vi "Pose_Create.vi"(9 "Heading":dbl, 10 "Y":dbl, 11 "X":dbl) -> (3 "out POSe":T1)   [LabVIEW 2019, in "PathExecution_Library.lvlib"]
uses:
  PathExecution_Library.lvlib
  POSE.ctl
  TRANSLATION.ctl
  ROTATION.ctl
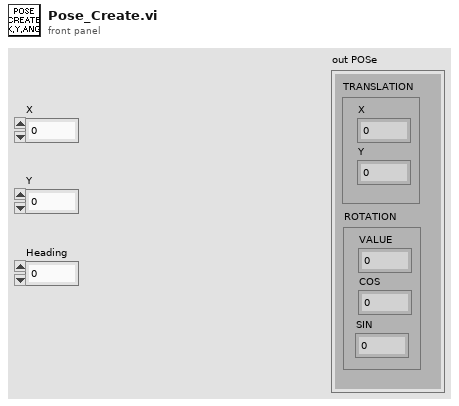
[diagram p1: front panel]
types:
  T1 = typedef "PathExecution_Library.lvlib/POSE.ctl" = cluster{"TRANSLATION":T2, "ROTATION":T3}
  T2 = typedef "PathExecution_Library.lvlib/TRANSLATION.ctl" = cluster{"X":dbl, "Y":dbl}
  T3 = typedef "PathExecution_Library.lvlib/ROTATION.ctl" = cluster{"VALUE":dbl, "COS":dbl, "SIN":dbl}
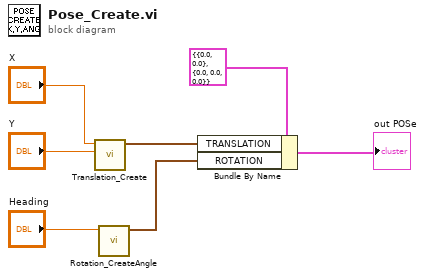
[diagram p0: block diagram]
diagram:
  n1 = call "Translation_Create.vi"("Y"="Y", "X"="X") -> ("TRANSLATION"=w3:T2)  [unwired: 9 in]
  n2 = call "Rotation_CreateAngle.vi"("Angle"="Heading") -> ("ROTATION"=w4:T3)  [unwired: 10 in]
  n3 = Bundle By Name(cluster=T1 {"TRANSLATION"={"X"=0.0, "Y"=0.0}, "ROTATION"={"VALUE"=0.0, "COS"=0.0, "SIN"=0.0}} ("sumPOSE"), "TRANSLATION"=w3, "ROTATION"=w4) -> (→"out POSe":T1)
